vi "SelectLengthsOfParts.vi"(8 "error in (no error)":errorcluster, 11 "reference in":refnum<class "Manipulator.lvclass">) -> (0 "error out":errorcluster, 3 "reference out":refnum<class "Manipulator.lvclass">)   [LabVIEW 2014, in "Manipulator.lvclass"]
uses:
  Manipulator.lvclass
panel:
  out "cok?":bool=TRUE
  out "bok?":bool=TRUE
  out "aok?":bool=TRUE
  in  "Accept Points":bool
  in  "c":dbl=100.0 caption="c ="
  in  "b":dbl=250.0 caption="b ="
  in  "a":dbl=250.0 caption="a ="
  # "[mm]"
  # "[mm]"
  # "[mm]"
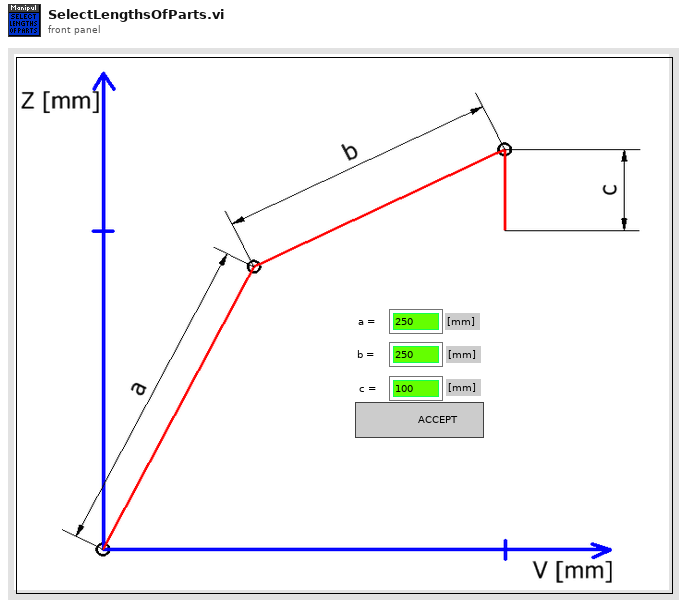
[diagram p1: front panel]
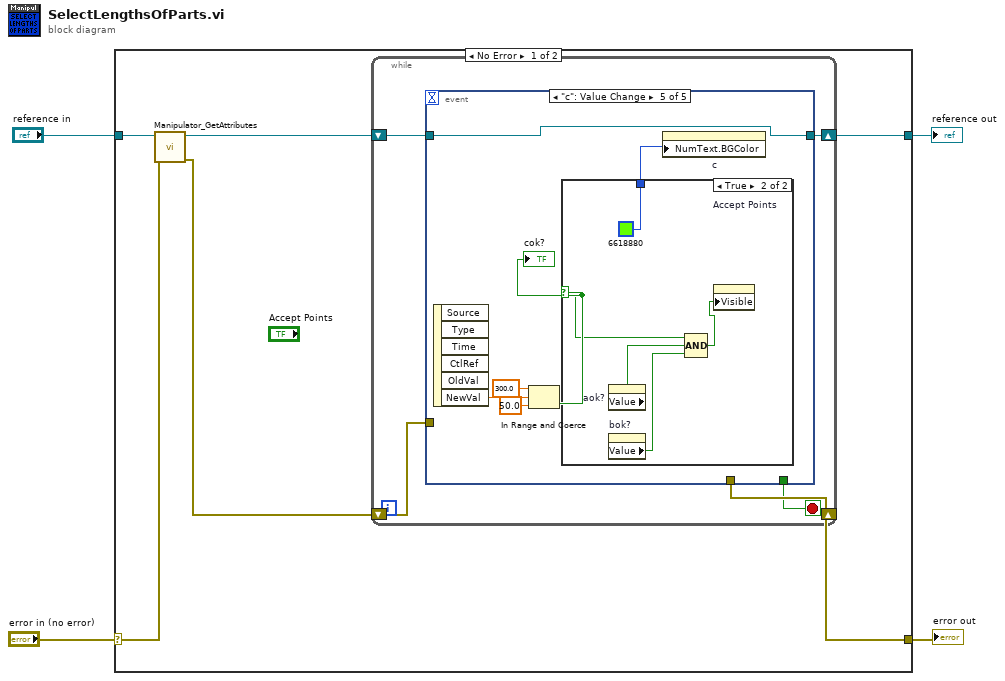
[diagram p0: block diagram]
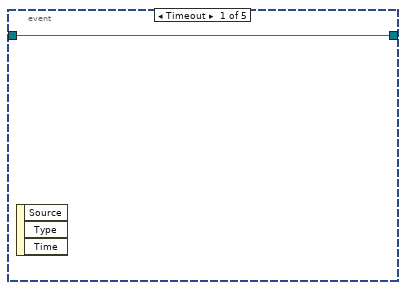
[diagram p2: hidden frame]
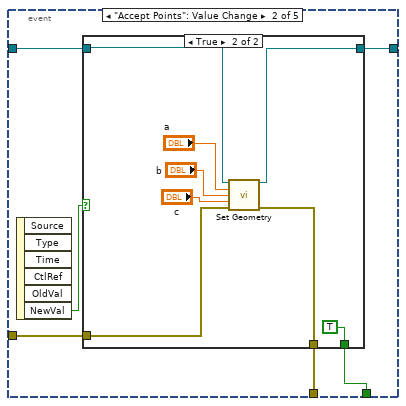
[diagram p3: hidden frame]
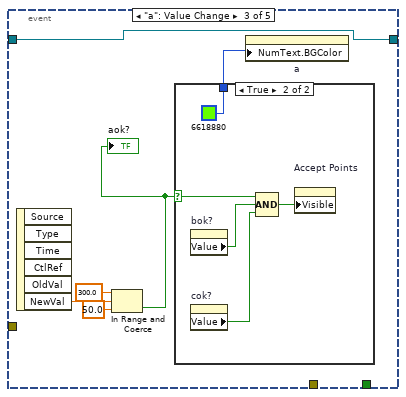
[diagram p5: hidden frame]
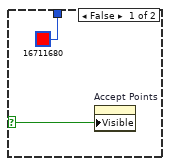
[diagram p6: hidden frame]
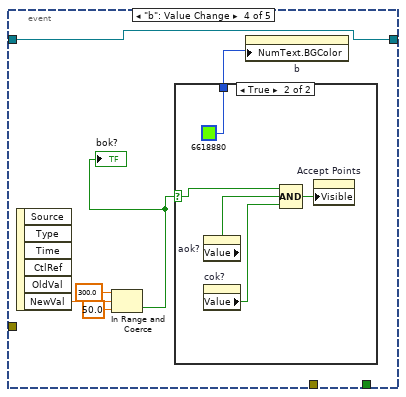
[diagram p7: hidden frame]
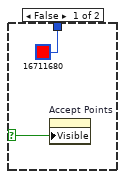
[diagram p8: hidden frame]
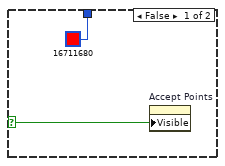
[diagram p9: hidden frame]
diagram:
  n1 = case shown="No Error" "error in (no error)" {
    selector: "error in (no error)" -> [w10 w72]
    tunnel: [w5 w72] -> w3
    tunnel: [w7 w71] -> w1
    tunnel: "reference in" -> [w9 w71]
    frame No Error {
      n2 = call "Manipulator_GetAttributes.vi"("error in (no error)"=w10, "reference in"=w9) -> ("error out"=w6:errorcluster, "reference out"=w8:refnum<class "Manipulator.lvclass">)  [unwired: 6 in, 2 out]
      n3 = while {
        shift-right: [w14] -> w7
        shift-left: w8 -> [w15]
        shift-right: [w12] -> w5
        shift-left: w6 -> [w13]
        stop <- w11 stop-if-true
        n4 = event shown="[4] \"c\": Value Change" {
          selector: _ -> [_ _ _ _ _]
          dyn-events: _ -> [_ _ _ _ _]
          timeout: _ -> [_ _ _ _ _]
          tunnel: w15 -> [w16 w21 w33 w46 w59]
          tunnel: [w16 w20 w33 w46 w59] -> w14
          tunnel: w13 -> [_ w19 _ _ _]
          tunnel: [_ w18 _ _ _] -> w12
          tunnel: [_ w17 _ _ _] -> w11
          event Timeout {
            n5 = event-data() -> ()  [unwired: 1 in, 3 out]
          }
          event "Accept Points": Value Change {
            n6 = event-data() -> ("NewVal"=w22:bool)  [unwired: 1 in, 5 out]
            n7 = case shown="True" w22 {
              tunnel: w21 -> [w23 w30]
              tunnel: [w23 w29] -> w20
              tunnel: w19 -> [_ w28]
              tunnel: [_ w27] -> w18
              tunnel: [_ TRUE] -> w17
              frame False {
              }
              frame True {
                n8 = call-dynamic "Set Geometry.vi"("reference in"=w30, "Lengths.a"="a", "Lengths.b"="b", "Lengths.c"="c", "error in (no error)"=w28) -> ("reference out"=w29:refnum<class "Manipulator.lvclass">, "error out"=w27:errorcluster)  [unwired: 9 in]
              }
            }
          }
          event "a": Value Change {
            n9 = event-data() -> ("NewVal"=w37:dbl)  [unwired: 1 in, 5 out]
            n10 = In Range and Coerce(upper limit=300.0, x=w37, lower limit=50.0) -> (In Range?=w32:bool)  [unwired: 1 out]
            "aok?" <- w32
            n11 = case shown="True" w32 {
              selector: w32 -> [w38 w41]
              tunnel: [u32 16711680 u32 6618880] -> w34
              frame False {
                n12 = property on="Accept Points" class="Bool"("Visible"=w38) -> ()  [unwired: 2 in, 2 out]
              }
              frame True {
                n13 = property on="bok?" class="Bool (strict)"() -> ("Value"=w43:bool)  [unwired: 2 in, 2 out]
                n14 = property on="cok?" class="Bool (strict)"() -> ("Value"=w40:bool)  [unwired: 2 in, 2 out]
                n15 = Compound Arithmetic op=AND(w41, w43, w40) -> (w42:bool)
                n16 = property on="Accept Points" class="Bool"("Visible"=w42) -> ()  [unwired: 2 in, 2 out]
              }
            }
            n17 = property on="a" class="DigNum (strict)"("NumText.BGColor"=w34) -> ()  [unwired: 2 in, 2 out]
          }
          event "b": Value Change {
            n18 = event-data() -> ("NewVal"=w50:dbl)  [unwired: 1 in, 5 out]
            n19 = In Range and Coerce(upper limit=300.0, x=w50, lower limit=50.0) -> (In Range?=w45:bool)  [unwired: 1 out]
            "bok?" <- w45
            n20 = case shown="True" w45 {
              selector: w45 -> [w51 w54]
              tunnel: [u32 16711680 u32 6618880] -> w47
              frame False {
                n21 = property on="Accept Points" class="Bool"("Visible"=w51) -> ()  [unwired: 2 in, 2 out]
              }
              frame True {
                n22 = property on="aok?" class="Bool (strict)"() -> ("Value"=w56:bool)  [unwired: 2 in, 2 out]
                n23 = property on="cok?" class="Bool (strict)"() -> ("Value"=w53:bool)  [unwired: 2 in, 2 out]
                n24 = Compound Arithmetic op=AND(w54, w56, w53) -> (w55:bool)
                n25 = property on="Accept Points" class="Bool"("Visible"=w55) -> ()  [unwired: 2 in, 2 out]
              }
            }
            n26 = property on="b" class="DigNum (strict)"("NumText.BGColor"=w47) -> ()  [unwired: 2 in, 2 out]
          }
          event "c": Value Change {
            n27 = event-data() -> ("NewVal"=w63:dbl)  [unwired: 1 in, 5 out]
            n28 = In Range and Coerce(upper limit=300.0, x=w63, lower limit=50.0) -> (In Range?=w58:bool)  [unwired: 1 out]
            "cok?" <- w58
            n29 = case shown="True" w58 {
              selector: w58 -> [w64 w67]
              tunnel: [u32 16711680 u32 6618880] -> w60
              frame False {
                n30 = property on="Accept Points" class="Bool"("Visible"=w64) -> ()  [unwired: 2 in, 2 out]
              }
              frame True {
                n31 = property on="aok?" class="Bool (strict)"() -> ("Value"=w69:bool)  [unwired: 2 in, 2 out]
                n32 = property on="bok?" class="Bool (strict)"() -> ("Value"=w68:bool)  [unwired: 2 in, 2 out]
                n33 = Compound Arithmetic op=AND(w67, w69, w68) -> (w66:bool)
                n34 = property on="Accept Points" class="Bool"("Visible"=w66) -> ()  [unwired: 2 in, 2 out]
              }
            }
            n35 = property on="c" class="DigNum (strict)"("NumText.BGColor"=w60) -> ()  [unwired: 2 in, 2 out]
          }
        }
      }
    }
    frame Error {
    }
  }
  "error out" <- w3
  "reference out" <- w1
